vi "GetRelatedPropertyByConnectedProperty.vi"(0 "Caps":T1, 1 "PropertyName":string="NI.Scratchpad64.I64", 5 "error in (no error)":errorcluster) -> (14 "Find?":bool, 15 "index of register":i32, 16 "The Register":T4, 19 "error out":errorcluster)   [LabVIEW 2018]
uses:
  Ctrl/Register.ctl
  Ctrl/Bitfield.ctl
  Ctrl/Caps.ctl
  Ctrl/Property.ctl
  Ctrl/PhysicalChannel.ctl
  Ctrl/Scale.ctl
  Ctrl/ScaleType.ctl
  Ctrl/Enum.ctl
  Ctrl/EnumValue.ctl
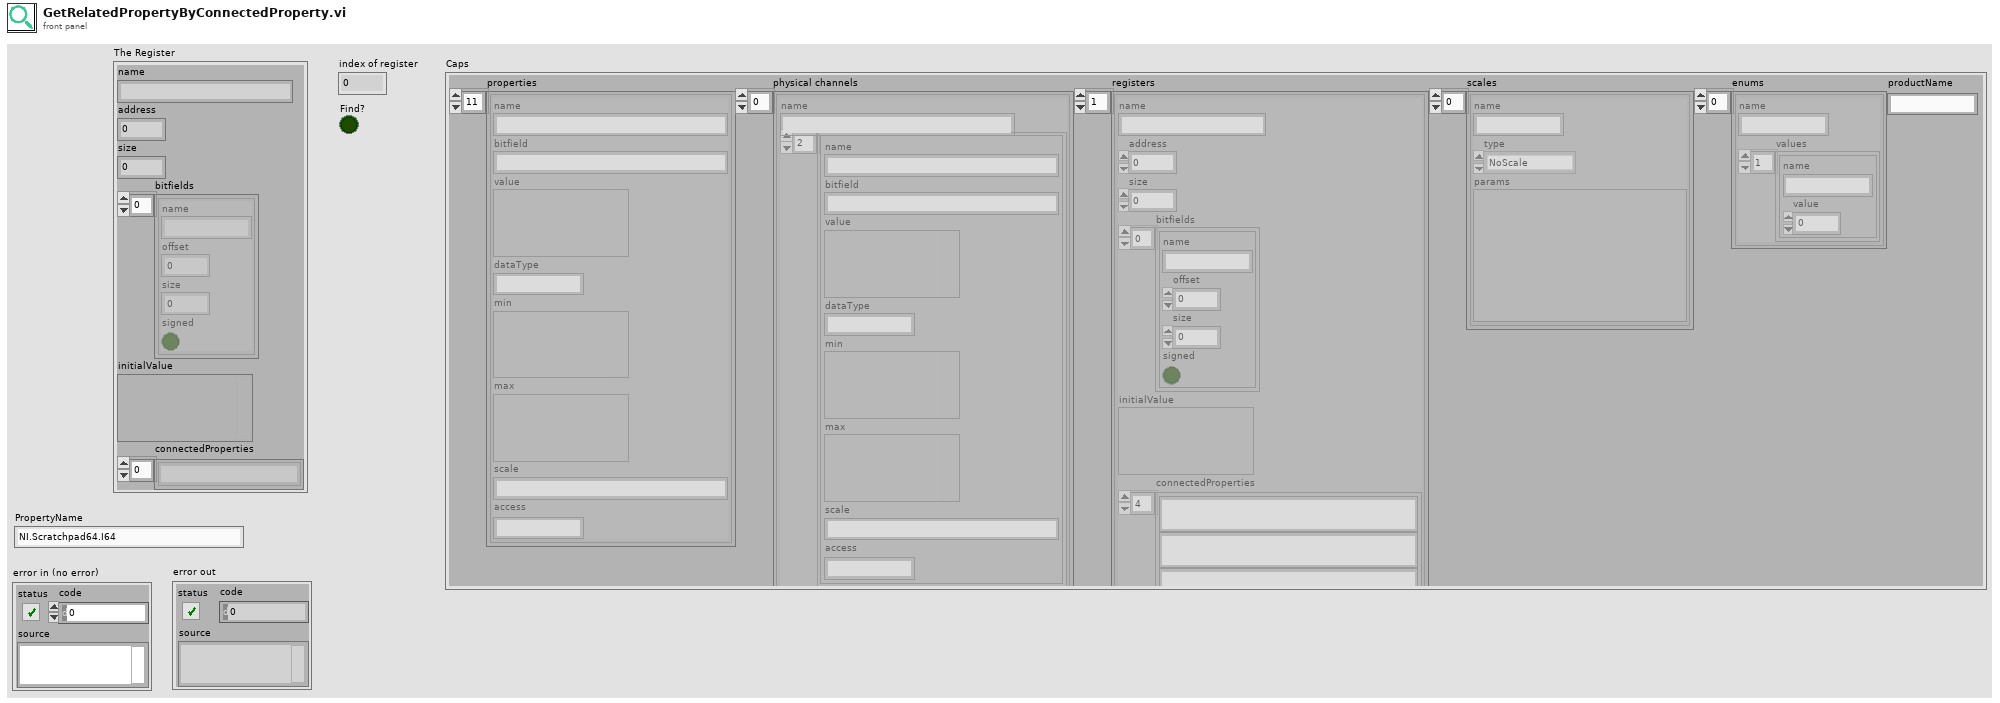
[diagram p1: front panel]
types:
  T1 = typedef "Caps.ctl" = cluster{"properties":T2[], "physical channels":T3[], "registers":T4[], "scales":T6[], "enums":T8[], "productName":string}
  T2 = typedef "Property.ctl" = cluster{"name":string, "bitfield":string, "value":variant, "dataType":string, "min":variant, "max":variant, "scale":string, "access":string}
  T3 = typedef "PhysicalChannel.ctl" = cluster{"name":string, "properties":T2[]}
  T4 = typedef "Register.ctl" = cluster{"name":string, "address":i32, "size":i32, "bitfields":T5[], "initialValue":variant, "connectedProperties":string[]}
  T5 = typedef "Bitfield.ctl" = cluster{"name":string, "offset":i32, "size":i32, "signed":bool}
  T6 = typedef "Scale.ctl" = cluster{"name":string, "type":T7, "params":variant}
  T7 = typedef "ScaleType.ctl" = enum16{"NoScale", "Table", "Polynomial", "Linear"}
  T8 = typedef "Enum.ctl" = cluster{"name":string, "values":T9[]}
  T9 = typedef "EnumValue.ctl" = cluster{"name":string, "value":i32}
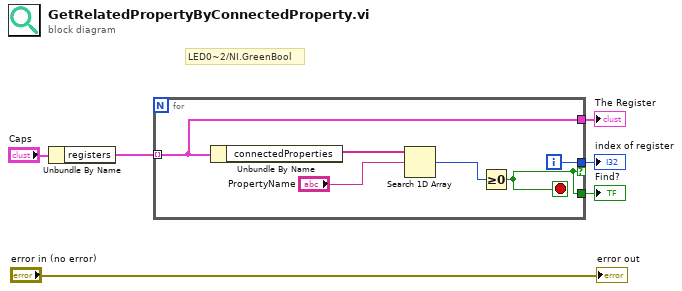
[diagram p0: block diagram]
diagram:
  # "LED0~2/NI.GreenBool"
  n1 = Unbundle By Name("Caps") -> ("registers"=w3:T4[])
  n2 = for {
    tunnel: w3 -> [w9] mode=indexing
    tunnel: [w8] -> w4 if=w7
    tunnel: [w9] -> w5
    tunnel: [w7] -> w6
    i -> [w8]
    stop <- w7 stop-if-true
    n3 = Unbundle By Name(w9) -> ("connectedProperties"=w12:string[])
    n4 = Search 1D Array(1D array=w12, element="PropertyName") -> (index of element=w10:i32)  [unwired: 1 in]
    n5 = Greater Or Equal To 0?(x=w10) -> (x >= 0?=w7:bool)
  }
  "index of register" <- w4
  "The Register" <- w5
  "Find?" <- w6
  "error out" <- "error in (no error)"
